vi "Next Sequence Filename.vi"(10 "Base path":path) -> (2 "Next Index":i32)   [LabVIEW 2023]
uses:
  <vilib>/regexp/Match Regular Expression.xnode
panel:
  out "Existing Files":string[](array[string])
  out "File Indices":i32[](array[numeric])
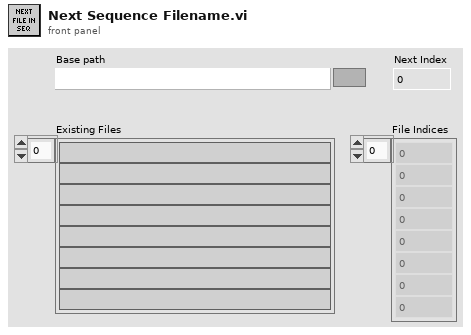
[diagram p1: front panel]
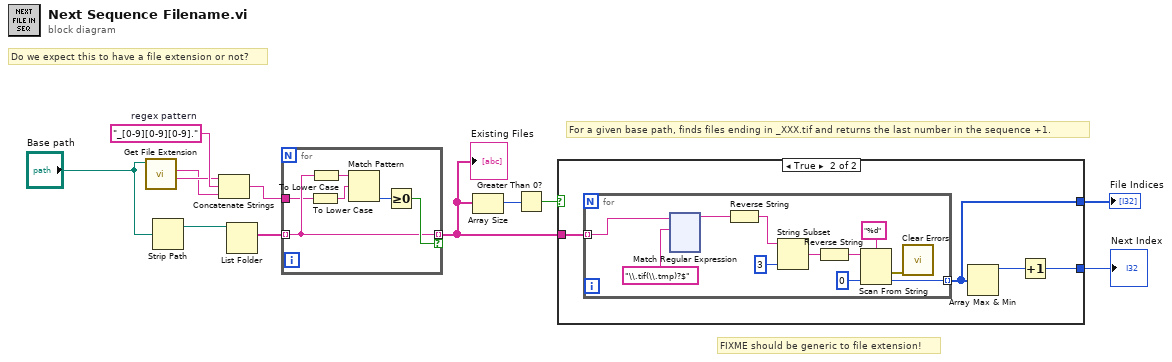
[diagram p0: block diagram]
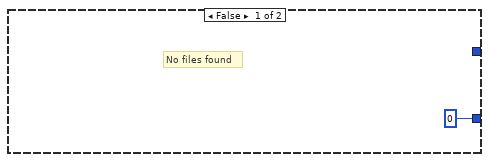
[diagram p2: hidden frame]
diagram:
  w10 = "_[0-9][0-9][0-9]."  # regex pattern
  # "FIXME should be generic to file extension!"
  # "Do we expect this to have a file extension or not?"
  # "For a given base path, finds files ending in _XXX.tif and returns the last number in the sequence +1."
  n1 = call <vilib>:"Get File Extension.vi"("file"="Base path") -> ("filename without extension"=w8:string, "lowercase file extension"=w7:string)  [unwired: 6 in, 3 out]
  n2 = Strip Path(path="Base path") -> (stripped path=w6:path)  [unwired: 1 out]
  n3 = Concatenate Strings(w8, w10, w7) -> (w9:string)
  n4 = List Folder(path=w6) -> (filenames=w11:string[])  [unwired: 3 in, 3 out]
  n5 = for {
    tunnel: w11 -> [w15] mode=indexing
    tunnel: w9 -> [w13]
    tunnel: [w15] -> w4 mode=indexing if=w17
    n6 = To Lower Case(string=w13) -> (all lower case string=w14:string)
    n7 = To Lower Case(string=w15) -> (all lower case string=w16:string)
    n8 = Match Pattern(string=w16, regular expression=w14) -> (offset past match=w18:i32)  [unwired: 1 in, 3 out]
    n9 = Greater Or Equal To 0?(x=w18) -> (x >= 0?=w17:bool)
  }
  "Existing Files" <- w4
  n10 = Array Size(array=w4) -> (size(s)=w2:i32)
  n11 = Greater Than 0?(x=w2) -> (x > 0?=w3:bool)
  n12 = case shown="True" w3 {
    tunnel: [0 w23] -> w5
    tunnel: w4 -> [_ w21]
    tunnel: [_ w20] -> w1
    frame False {
      # "No files found"
    }
    frame True {
      n13 = for {
        tunnel: [w32] -> w20 mode=indexing
        tunnel: w21 -> [w24] mode=indexing
        n14 = xnode "Match Regular Expression"("input string"=w24, "regular expression"="\\.tif(\\.tmp)?$") -> ("before match"=w26:string)  [unwired: 4 in, 4 out]
        n15 = Reverse String(1:w26) -> (0:w30:string)
        n16 = String Subset(string=w30, length (rest)=3 ("length (rest)")) -> (substring=w29:string)  [unwired: 1 in]
        n17 = Reverse String(1:w29) -> (0:w28:string)
        n18 = Scan From String(format string="%d", input string=w28, default 1=0 ("default value 1")) -> (error out=w31:errorcluster, output 1=w32:i32)  [unwired: 2 in, 2 out]
        n19 = call <vilib>:"Clear Errors.vi"("error in (no error)"=w31) -> ()  [unwired: 5 in, 2 out]
      }
      n20 = Array Max & Min(array=w20) -> (max value=w22:i32)  [unwired: 3 out]
      n21 = Increment(x=w22) -> (x+1=w23:i32)
    }
  }
  "Next Index" <- w5
  "File Indices" <- w1
